vi "Main.vi"() -> ()   [LabVIEW 2015]
doc: "The myRIO Project template acquires acceleration data from the onboard accelerometer and displays the changes of acceleration values in a waveform chart."
uses:
  <vilib>/myRIO/Instrument Drivers/Onboard IO/DIO/typedefs/DIO Reference.ctl
  <vilib>/myRIO/Common/Instrument Driver Framework/Utilities/typedefs/myRIO Generic Hardware Reference.ctl
  <vilib>/myRIO/Common/Instrument Driver Framework/Utilities/typedefs/Hardware Version Enum.ctl
  <vilib>/myRIO/Common/Instrument Driver Framework/Utilities/typedefs/myRIO v1.0 Reference.ctl
  <vilib>/myRIO/Common/Instrument Driver Framework/Utilities/typedefs/Generic FPGA Reference.ctl
  <vilib>/myRIO/Common/Instrument Driver Framework/myRIO v1.0/DIO/typedefs/DIO Channels List.ctl
  <vilib>/myRIO/Common/Instrument Driver Framework/myRIO v1.0/DIO/typedefs/DIO Channels Enum.ctl
  <vilib>/userdefined/High Color/nirio_resource_hc.ctl
  <vilib>/myRIO/Instrument Drivers/Onboard IO/AI/typedefs/AI Reference.ctl
  <vilib>/myRIO/Common/Instrument Driver Framework/myRIO v1.0/AI/typedefs/AI Channels List.ctl
  <vilib>/myRIO/Common/Instrument Driver Framework/myRIO v1.0/AI/typedefs/AI Channels Enum.ctl
  <vilib>/myRIO/Common/Instrument Driver Framework/Utilities/typedefs/Analog Scaling Constants List.ctl
  <vilib>/myRIO/Common/Instrument Driver Framework/Utilities/typedefs/Analog Scaling Constants.ctl
  <vilib>/myRIO/Instrument Drivers/Onboard IO/PWM/typedefs/PWM Reference.ctl
  <vilib>/myRIO/Common/Instrument Driver Framework/myRIO v1.0/PWM/typedefs/PWM Channels Enum.ctl
  <vilib>/myRIO/Instrument Drivers/Onboard IO/PWM/typedefs/PWM Configuration.ctl
  <vilib>/myRIO/Instrument Drivers/Onboard Devices/Accelerometer/typedefs/Accelerometer Reference.ctl
  <vilib>/myRIO/Common/Instrument Driver Framework/myRIO v1.0/Accelerometer/typedefs/Accelerometer Channels List.ctl
  <vilib>/myRIO/Common/Instrument Driver Framework/myRIO v1.0/Accelerometer/typedefs/Accelerometer Channels Enum.ctl
  <vilib>/myRIO/Common/Instrument Driver Framework/Utilities/vis/Is FPGA Ref Available.vi
  <vilib>/myRIO/Common/Instrument Driver Framework/myRIO v1.0/AI/vis/myRIO v1.1 Open AI.vi
  <vilib>/myRIO/Instrument Drivers/Onboard IO/AI/vis/Read.vi
  <vilib>/myRIO/Common/Instrument Driver Framework/myRIO v1.0/DIO/vis/myRIO v1.1 Open DIO.vi
  <vilib>/myRIO/Instrument Drivers/Onboard IO/DIO/vis/Read.vi
  <vilib>/myRIO/Instrument Drivers/Onboard IO/DIO/vis/Write.vi
  <vilib>/myRIO/Common/Instrument Driver Framework/myRIO v1.0/PWM/vis/myRIO v1.1 Open PWM.vi
  <vilib>/myRIO/Instrument Drivers/Onboard IO/PWM/vis/Set Duty Cycle and Frequency.vi
  <vilib>/myRIO/Common/Instrument Driver Framework/myRIO v1.0/Accelerometer/vis/myRIO v1.1 Open Accelerometer.vi
  <vilib>/myRIO/Instrument Drivers/Onboard Devices/Accelerometer/vis/Read.vi
  <vilib>/myRIO/Common/Instrument Driver Framework/Utilities/vis/Validate Channels.vi
  <vilib>/myRIO/Common/Instrument Driver Framework/myRIO v1.0/AI/vis/myRIO v1.0 Reserve AI.vi
  <vilib>/myRIO/Common/Instrument Driver Framework/myRIO v1.0/DIO/vis/myRIO v1.0 Reserve DIO.vi
  <vilib>/myRIO/Common/Instrument Driver Framework/myRIO v1.0/PWM/vis/myRIO v1.0 Reserve PWM.vi
  <vilib>/myRIO/Common/Instrument Driver Framework/myRIO v1.0/Accelerometer/vis/myRIO v1.0 Reserve Accelerometer.vi
  <vilib>/myRIO/Common/Instrument Driver Framework/myRIO v1.0/UART/vis/myRIO v1.0 Close UART.vi
  <vilib>/myRIO/Common/Instrument Driver Framework/myRIO v1.0/AI/vis/myRIO v1.0 Build MUX Configuration AI.vi
  <vilib>/myRIO/Common/Instrument Driver Framework/myRIO v1.0/Resource Manager/vis/myRIO v1.0 Reserve Channel List.vi
  <vilib>/myRIO/Common/Instrument Driver Framework/myRIO v1.0/DIO/vis/myRIO v1.0 Build MUX Configuration DIO.vi
  <vilib>/myRIO/Common/Instrument Driver Framework/myRIO v1.0/PWM/vis/myRIO v1.0 Build MUX Configuration PWM.vi
  <vilib>/myRIO/Common/Instrument Driver Framework/myRIO v1.0/Accelerometer/vis/myRIO v1.0 Build MUX Configuration Accelerometer.vi
  <vilib>/myRIO/Common/Instrument Driver Framework/myRIO v1.0/Resource Manager/vis/myRIO v1.0 Reserve Channel.vi
  <vilib>/myRIO/Common/Instrument Driver Framework/myRIO v1.0/Resource Manager/vis/myRIO v1.0 Unreserve Channel.vi
  <vilib>/myRIO/Common/Instrument Driver Framework/myRIO v1.0/Resource Manager/vis/myRIO v1.0 Create Configuration List.vi
  <vilib>/myRIO/Common/Instrument Driver Framework/myRIO v1.0/Resource Manager/vis/myRIO v1.0 Build Mutex Name.vi
  <vilib>/Utility/VariantDataType/GetNumericInfo.vi
  <vilib>/Utility/error.llb/Error Cluster From Error Code.vi
  <vilib>/myRIO/Common/Instrument Driver Framework/myRIO v1.0/myRIO v1.1 Open.vi
  <vilib>/myRIO/Common/Instrument Driver Framework/Utilities/vis/IO Manager.vi
  <vilib>/myRIO/Common/Instrument Driver Framework/Utilities/vis/Configuration Manager.vi
  <vilib>/myRIO/Common/Instrument Driver Framework/myRIO v1.0/Resource Manager/vis/myRIO v1.0 Configure IO.vi
  <vilib>/myRIO/Common/Instrument Driver Framework/myRIO v1.0/myRIO v1.0 Close.vi
  <vilib>/myRIO/Common/Instrument Driver Framework/myRIO v1.0/DIO/vis/myRIO v1.0 Read DIO.vi
  <vilib>/myRIO/Common/Instrument Driver Framework/myRIO v1.0/AI/vis/myRIO v1.0 Get Scaling Constants AI.vi
  <vilib>/myRIO/Common/Instrument Driver Framework/myRIO v1.0/AI/vis/myRIO v1.0 Read AI.vi
  <vilib>/myRIO/Common/Instrument Driver Framework/myRIO v1.0/PWM/vis/myRIO v1.0 Write PWM.vi
  <vilib>/myRIO/Common/Instrument Driver Framework/myRIO v1.0/DIO/vis/myRIO v1.0 Write DIO.vi
  <vilib>/myRIO/Common/Instrument Driver Framework/myRIO v1.0/Accelerometer/vis/myRIO v1.0 Get Scaling Constant Accelerometer.vi
  <vilib>/myRIO/Common/Instrument Driver Framework/myRIO v1.0/Accelerometer/vis/myRIO v1.0 Read Accelerometer.vi
  <vilib>/myRIO/Common/Instrument Driver Framework/Utilities/vis/FPGA Ref Manager.vi
  <vilib>/myRIO/Common/Instrument Driver Framework/myRIO v1.0/myRIO v1.0 Reset FPGA.vi
  <vilib>/myRIO/Common/Instrument Driver Framework/myRIO v1.0/IRQ/vis/myRIO v1.0 IRQ Info FGV.vi
  <vilib>/myRIO/Common/Instrument Driver Framework/myRIO v1.0/IRQ/vis/myRIO v1.0 Timer IRQ Info FGV.vi
  <vilib>/myRIO/Common/Instrument Driver Framework/myRIO v1.0/IRQ/vis/myRIO v1.0 ISR Agent.vi
  <vilib>/myRIO/Express VI/Onboard IO/DI/DI Express VI.xnode
  <vilib>/myRIO/Instrument Drivers/Onboard IO/DIO/vis/myRIO DIO Open.xnode
  <vilib>/myRIO/Express VI/Onboard IO/AI/AI Express VI.xnode
  <vilib>/myRIO/Instrument Drivers/Onboard IO/AI/vis/myRIO AI Open.xnode
  <vilib>/myRIO/Express VI/Onboard IO/PWM/PWM Express VI.xnode
  <vilib>/myRIO/Instrument Drivers/Onboard IO/PWM/vis/myRIO PWM Open.xnode
  <vilib>/myRIO/Express VI/Onboard IO/DO/DO Express VI.xnode
  <vilib>/myRIO/Express VI/Onboard Devices/Accelerometer/Accelerometer Express VI.xnode
  <vilib>/myRIO/Instrument Drivers/Onboard Devices/Accelerometer/vis/myRIO Accelerometer Open.xnode
  <vilib>/myRIO/Instrument Drivers/Utilities/Utilities.lvlib
  <vilib>/myRIO/Instrument Drivers/Onboard Devices/Accelerometer/Accelerometer.lvlib
  <vilib>/myRIO/Instrument Drivers/Onboard IO/PWM/PWM.lvlib
  <vilib>/myRIO/Instrument Drivers/Onboard IO/DIO/DIO.lvlib
  <vilib>/myRIO/Instrument Drivers/Onboard IO/AI/AI.lvlib
panel:
  out "Acceleration":T1(graph)
  out "error out":errorcluster
  in  "Stop":bool
  # "Overview: The myRIO Project template acquires acceleration data from the onboard accelerometer and displays the changes of acceleration values in a waveform chart.\nInstructions:\n1. Check the myRIO target IP address in the project and make sure the target IP address is correct. \n2. Run this VI."
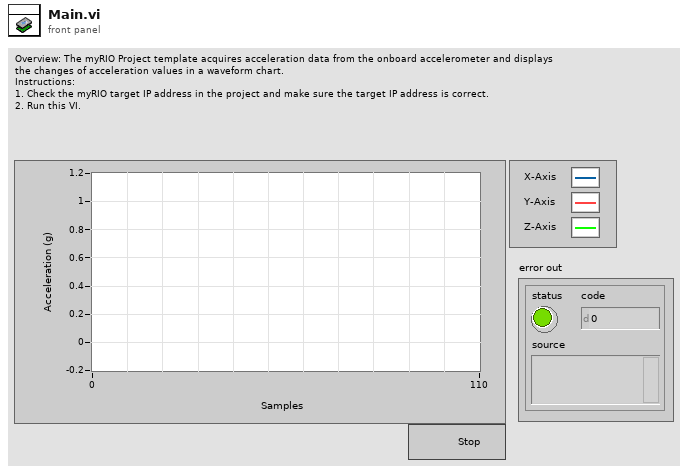
[diagram p1: front panel]
types:
  T1 = cluster{"X-Axis":dbl, "Y-Axis":dbl, "Z-Axis":dbl}
  T2 = typedef "AI.lvlib/AI Reference.ctl" = cluster{"myRIO Reference":T3, "AI Channels List":T7, "AI Scaling Constants List":T9}
  T3 = typedef "myRIO Generic Hardware Reference.ctl" = cluster{"myRIO Model":T4, "myRIO Hardware Reference":T5}
  T4 = typedef "Hardware Version Enum.ctl" = enum16{"Unknown", "myRIO-1900", "myRIO-1950", "roboRIO"}
  T5 = typedef "myRIO v1.0 Reference.ctl" = cluster{"Generic FPGA Reference":T6, "Allow multiple opens":bool}
  T6 = typedef "Generic FPGA Reference.ctl" = refnum<k20>
  T7 = typedef "AI Channels List.ctl" = T8[]
  T8 = typedef "AI Channels Enum.ctl" = enum16{"Not Connected", "AudioIn/Left", "AudioIn/Right", "C/AI0", "C/AI1", "A/AI0", "A/AI1", "A/AI2", "A/AI3", "B/AI0", "B/AI1", "B/AI2", "B/AI3", "AI/AI0", "AI/AI1", "AI/AI2", "AI/AI3"}
  T9 = typedef "Analog Scaling Constants List.ctl" = T10[]
  T10 = typedef "Analog Scaling Constants.ctl" = cluster{"LSB Weight (Volts)":dbl, "Offset (Volts)":dbl, "Signed?":bool}
  T11 = typedef "nirio_resource_hc.ctl" = tag
  T12 = typedef "DIO.lvlib/DIO Reference.ctl" = cluster{"myRIO Reference":T3, "DIO Channels List":T13}
  T13 = typedef "DIO Channels List.ctl" = T14[]
  T14 = typedef "DIO Channels Enum.ctl" = enum16{"Not Connected", "C/DIO0", "C/DIO1", "C/DIO2", "C/DIO3", "C/DIO4", "C/DIO5", "C/DIO6", "C/DIO7", "A/DIO0", "A/DIO1", "A/DIO2", "A/DIO3", "A/DIO4", "A/DIO5", "A/DIO6", "A/DIO7", "A/DIO8", "A/DIO9", "A/DIO10", "A/DIO11", "A/DIO12", "A/DIO13", "A/DIO14", "A/DIO15", "B/DIO0", "B/DIO1", "B/DIO2", "B/DIO3", "B/DIO4", "B/DIO5", "B/DIO6", "B/DIO7", "B/DIO8", "B/DIO9", "B/DIO10", "B/DIO11", "B/DIO12", "B/DIO13", "B/DIO14", "B/DIO15", "LED0", "LED1", "LED2", "LED3", "Button0", "DIO/DIO0", "DIO/DIO1", "DIO/DIO2", "DIO/DIO3", "DIO/DIO4", "DIO/DIO5", "DIO/DIO6", "DIO/DIO7", "DIO/DIO8", "DIO/DIO9", "SPI/CS0", "SPI/CS1", "SPI/CS2", "SPI/CS3", "LED RADIO (Green)", "LED RADIO (Red)", "LED COMM (Green)", "LED COMM (Red)", "LED MODE (Green)", "LED MODE (Red)"}
  T15 = typedef "PWM.lvlib/PWM Reference.ctl" = cluster{"myRIO Reference":T3, "PWM Channels Enum":T16, "PWM Configuration":T17}
  T16 = typedef "PWM Channels Enum.ctl" = enum16{"Not Connected", "C/PWM0", "C/PWM1", "A/PWM0", "A/PWM1", "A/PWM2", "B/PWM0", "B/PWM1", "B/PWM2", "PWM/PWM0", "PWM/PWM1", "PWM/PWM2", "PWM/PWM3", "PWM/PWM4", "PWM/PWM5", "PWM/PWM6", "PWM/PWM7", "PWM/PWM8", "PWM/PWM9"}
  T17 = typedef "PWM.lvlib/PWM Configuration.ctl" = cluster{"Frequency":dbl, "Duty Cycle":dbl}
  T18 = typedef "Accelerometer.lvlib/Accelerometer Reference.ctl" = cluster{"myRIO Reference":T3, "Accelerometer Channels List":T19, "LSB Weight":dbl}
  T19 = typedef "Accelerometer Channels List.ctl" = T20[]
  T20 = typedef "Accelerometer Channels Enum.ctl" = enum16{"Not Connected", "X-Axis", "Y-Axis", "Z-Axis"}
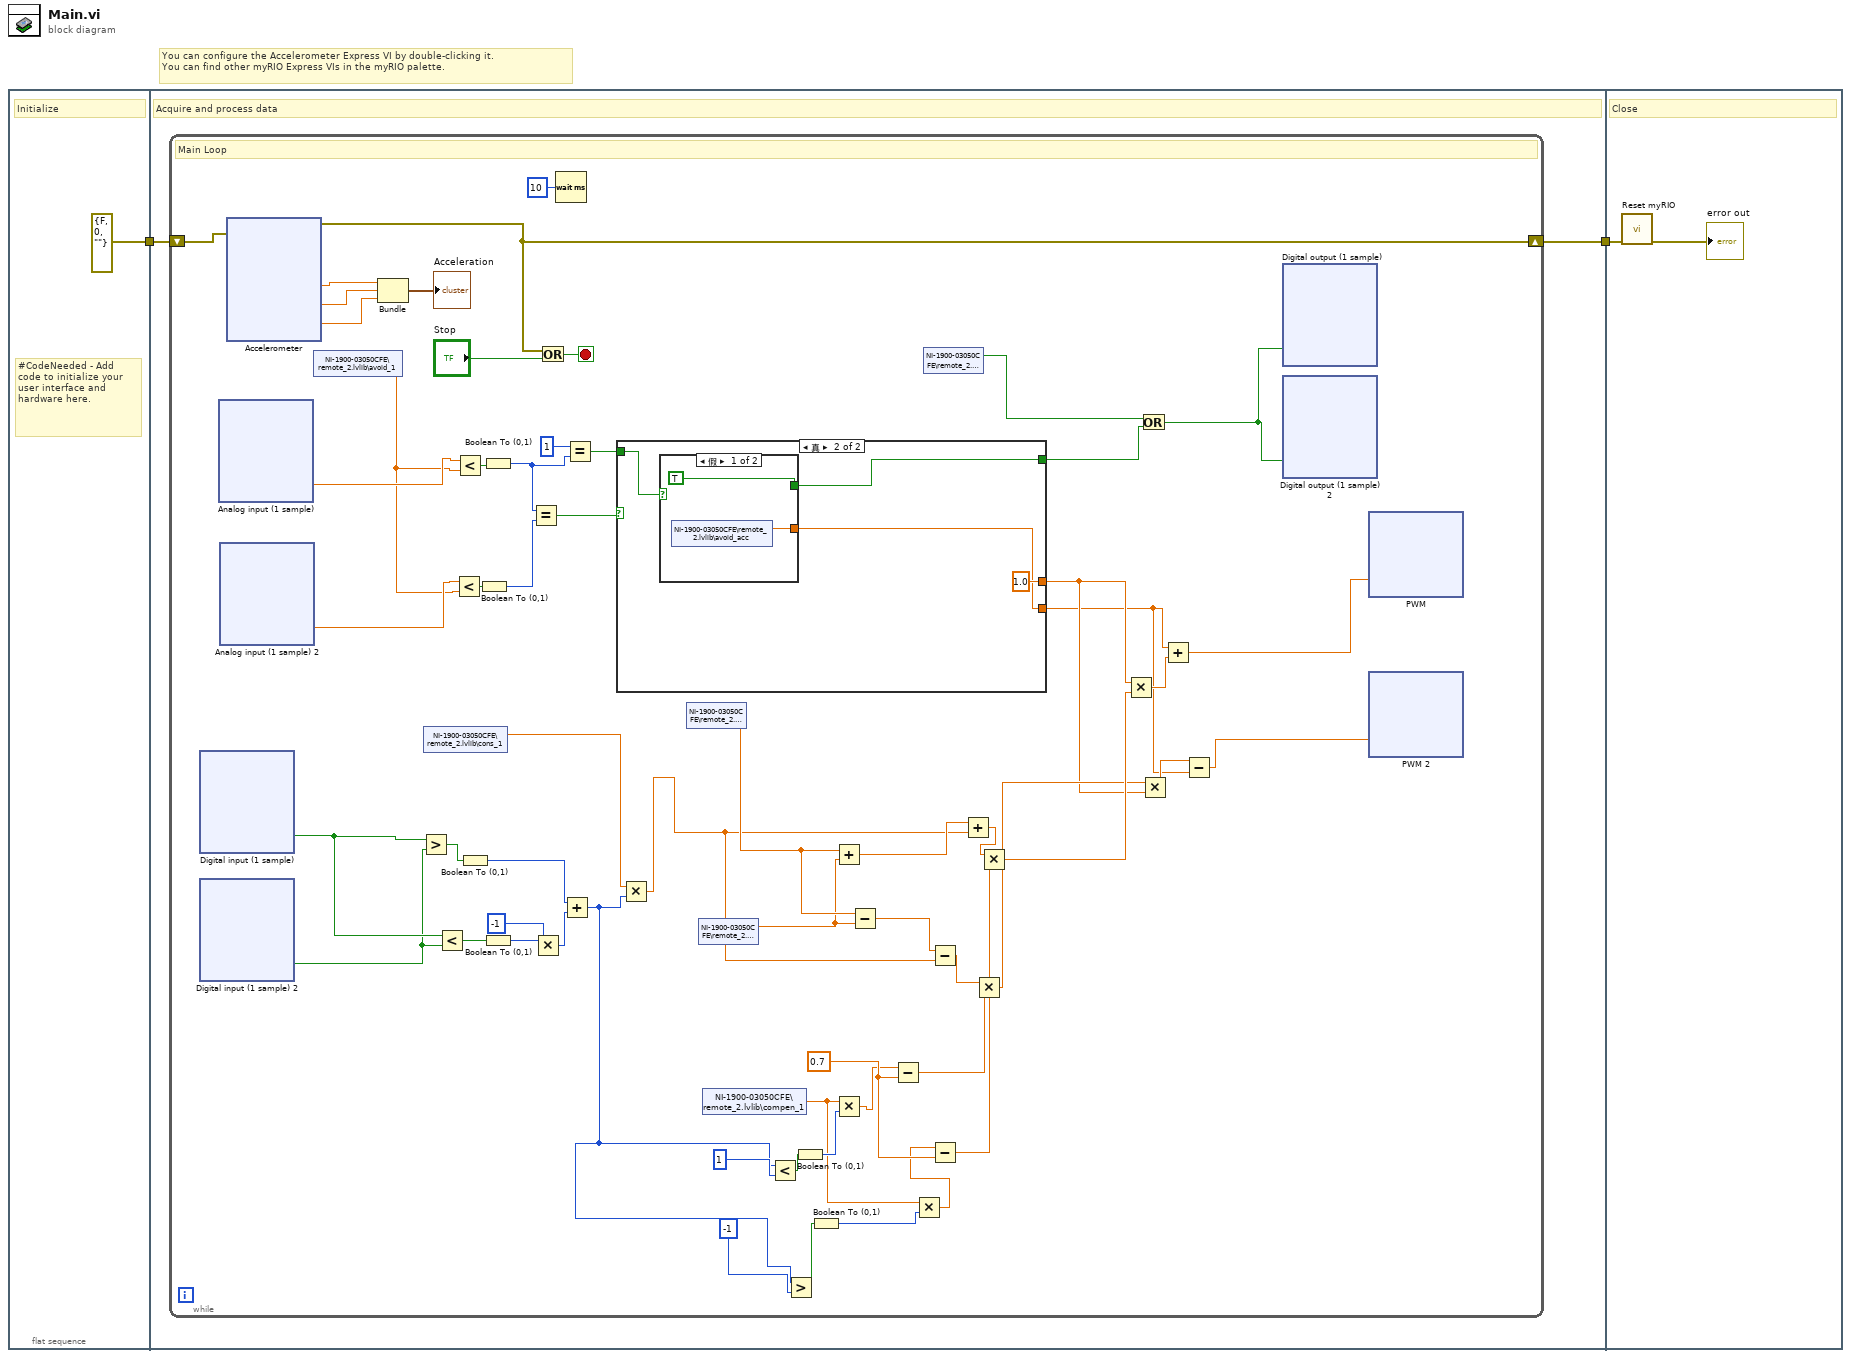
[diagram p0: block diagram]
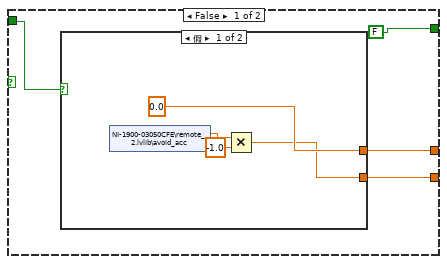
[diagram p2: hidden frame]
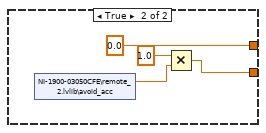
[diagram p3: hidden frame]
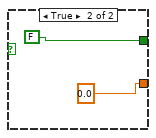
[diagram p4: hidden frame]
diagram:
  # "You can configure the Accelerometer Express VI by double-clicking it.\nYou can find other myRIO Express VIs in the myRIO palette."
  n1 = flat-sequence {
    tunnel: [errorcluster {"status"=FALSE, "code"=0, "source"=""} ("error in (no error)")] -> w2
    tunnel: w2 -> [w5]
    tunnel: [w4] -> w1
    tunnel: w1 -> [w409]
    frame #0 {
      # "#CodeNeeded - Add code to initialize your user interface and hardware here."
      # "Initialize"
    }
    frame #1 {
      # "Acquire and process data"
      n2 = while {
        shift-right: [w59] -> w4
        shift-left: w5 -> [w60]
        stop <- w63 stop-if-true
        w32 = 0.7 ("y")
        # "Main Loop"
        n3 = xnode "Digital input (1 sample)"() -> ("A/DIO2 (Pin 15)"=w50:bool)  [unwired: 1 in, 1 out]
        n4 = xnode "Digital input (1 sample) 2"() -> ("A/DIO3 (Pin 17)"=w49:bool)  [unwired: 1 in, 1 out]
        n5 = xnode "Analog input (1 sample)"() -> ("A/AI0 (Pin 3)"=w9:dbl)  [unwired: 1 in, 1 out]
        n6 = xnode "Analog input (1 sample) 2"() -> ("A/AI1 (Pin 5)"=w7:dbl)  [unwired: 1 in, 1 out]
        n7 = xnode "Accelerometer"("error in (no error)"=w60) -> ("X-Axis"=w58:dbl, "Y-Axis"=w57:dbl, "Z-Axis"=w56:dbl, "error out"=w59:errorcluster)
        n8 = shared-variable "NI-1900-03050CFE\\remote_2.lvlib\\avoid_1"() -> (w6:dbl)  [unwired: 1 in, 1 out]
        n9 = Bundle("X-Axis"=w58, "Y-Axis"=w57, "Z-Axis"=w56) -> (→"Acceleration":T1)  [unwired: 1 in]
        n10 = Greater?(x=w50, y=w49) -> (0:w51:bool)
        n11 = shared-variable "NI-1900-03050CFE\\remote_2.lvlib\\cons_1"() -> (w43:dbl)  [unwired: 1 in, 1 out]
        n12 = Less?(x=w50, y=w49) -> (x < y?=w48:bool)
        n13 = Less?(x=w7, y=w6) -> (x < y?=w8:bool)
        n14 = Less?(x=w9, y=w6) -> (x < y?=w10:bool)
        n15 = Boolean To (0,1)(Boolean=w51) -> (0, 1=w44:i16)
        n16 = Boolean To (0,1)(Boolean=w8) -> (0, 1=w26:i16)
        n17 = Boolean To (0,1)(Boolean=w10) -> (0, 1=w24:i16)
        n18 = Boolean To (0,1)(Boolean=w48) -> (0, 1=w47:i16)
        n19 = Equal?(x=w24, y=w26) -> (x = y?=w25:bool)
        n20 = Multiply(x=w47, y=i16 -1) -> (x*y=w45:i16)
        n21 = Or(x=w59, y="Stop") -> (x .or. y?=w63:bool)
        n22 = Wait (ms)(milliseconds to wait=u32 10) -> ()  [unwired: 1 out]
        n23 = Add(x=w44, y=w45) -> (x+y=w33:i16)
        n24 = Equal?(x=i16 1, y=w24) -> (x = y?=w22:bool)
        n25 = case shown="真" w25 {
          tunnel: w22 -> [w68 w80]
          tunnel: [FALSE ("y") w79] -> w20
          tunnel: [w66 1.0 ("x")] -> w15
          tunnel: [w65 w77] -> w12
          frame False {
            n26 = case shown="假" w68 {
              tunnel: [0.0 ("x") 0.0 ("x")] -> w66
              tunnel: [w69 w75] -> w65
              frame False {
                n27 = shared-variable "NI-1900-03050CFE\\remote_2.lvlib\\avoid_acc"() -> (w71:dbl)  [unwired: 1 in, 1 out]
                n28 = Multiply(x=w71, y=-1.0) -> (x*y=w69:dbl)
              }
              frame True {
                n29 = shared-variable "NI-1900-03050CFE\\remote_2.lvlib\\avoid_acc"() -> (w74:dbl)  [unwired: 1 in, 1 out]
                n30 = Multiply(x=1.0, y=w74) -> (x*y=w75:dbl)
              }
            }
          }
          frame True {
            n31 = case shown="假" w80 {
              tunnel: [TRUE ("y") FALSE ("y")] -> w79
              tunnel: [w81 0.0 ("x")] -> w77
              frame False {
                n32 = shared-variable "NI-1900-03050CFE\\remote_2.lvlib\\avoid_acc"() -> (w81:dbl)  [unwired: 1 in, 1 out]
              }
              frame True {
              }
            }
          }
        }
        n33 = Multiply(x=w43, y=w33) -> (x*y=w42:dbl)
        n34 = shared-variable "NI-1900-03050CFE\\remote_2.lvlib\\p1"() -> (w55:dbl)  [unwired: 1 in, 1 out]
        n35 = shared-variable "NI-1900-03050CFE\\remote_2.lvlib\\p2"() -> (w54:dbl)  [unwired: 1 in, 1 out]
        n36 = shared-variable "NI-1900-03050CFE\\remote_2.lvlib\\compen_1"() -> (w38:dbl)  [unwired: 1 in, 1 out]
        n37 = Less?(x=w33, y=i16 1) -> (x < y?=w37:bool)
        n38 = Greater?(x=w33, y=i16 -1) -> (0:w35:bool)
        n39 = Boolean To (0,1)(Boolean=w37) -> (0, 1=w39:i16)
        n40 = Boolean To (0,1)(Boolean=w35) -> (0, 1=w27:i16)
        n41 = Add(x=w55, y=w54) -> (x+y=w53:dbl)
        n42 = Multiply(x=w38, y=w39) -> (x*y=w31:dbl)
        n43 = Subtract(x=w55, y=w54) -> (x-y=w52:dbl)
        n44 = Subtract(x=w31, y=w32) -> (x-y=w30:dbl)
        n45 = Multiply(x=w38, y=w27) -> (x*y=w29:dbl)
        n46 = shared-variable "NI-1900-03050CFE\\remote_2.lvlib\\d1"() -> (w21:bool)  [unwired: 1 in, 1 out]
        n47 = Subtract(x=w52, y=w42) -> (x-y=w41:dbl)
        n48 = Subtract(x=w29, y=w32) -> (x-y=w28:dbl)
        n49 = Add(x=w53, y=w42) -> (x+y=w40:dbl)
        n50 = Multiply(x=w41, y=w30) -> (x*y=w16:dbl)
        n51 = Multiply(x=w40, y=w28) -> (x*y=w17:dbl)
        n52 = Multiply(x=w15, y=w17) -> (x*y=w14:dbl)
        n53 = Or(x=w21, y=w20) -> (x .or. y?=w19:bool)
        n54 = Multiply(x=w16, y=w15) -> (x*y=w13:dbl)
        n55 = Add(x=w12, y=w14) -> (x+y=w18:dbl)
        n56 = Subtract(x=w13, y=w12) -> (x-y=w11:dbl)
        n57 = xnode "Digital output (1 sample)"("A/DIO0 (Pin 11)"=w19) -> ()  [unwired: 1 in, 1 out]
        n58 = xnode "Digital output (1 sample) 2"("A/DIO1 (Pin 13)"=w19) -> ()  [unwired: 1 in, 1 out]
        n59 = xnode "PWM"("Duty Cycle"=w18) -> ()  [unwired: 1 in, 1 out]
        n60 = xnode "PWM 2"("Duty Cycle"=w11) -> ()  [unwired: 1 in, 1 out]
      }
    }
    frame #2 {
      # "Close"
      n61 = call <vilib>:"Reset myRIO.vi"("error in (no error)"=w409) -> ("error out"=→"error out":errorcluster)  [unwired: 10 in]
    }
  }
